vi "Case.vi"() -> ()   [LabVIEW 2013]
panel:
  out "Arbitary":bool
  out "Random":bool
  out "Sawtooth":bool
  out "Triangle":bool
  out "Square":bool
  out "Sine":bool
  in  "Triangle":bool
  in  "Random":bool
  in  "Arbitary":bool
  in  "Sine":bool
  in  "Square":bool
  in  "Sawtooth":bool
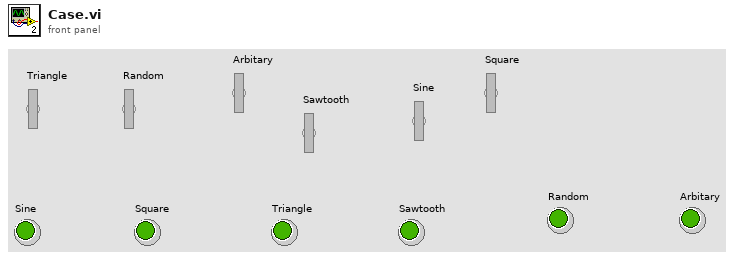
[diagram p1: front panel]
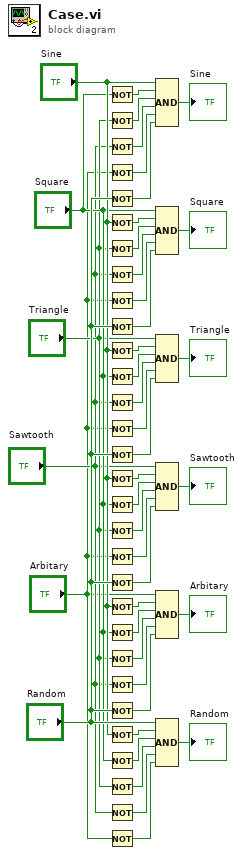
[diagram p0: block diagram]
diagram:
  n1 = Not(x="Square") -> (.not. x?=w42:bool)
  n2 = Not(x="Triangle") -> (.not. x?=w41:bool)
  n3 = Not(x="Sawtooth") -> (.not. x?=w40:bool)
  n4 = Not(x="Arbitary") -> (.not. x?=w39:bool)
  n5 = Not(x="Random") -> (.not. x?=w38:bool)
  n6 = Not(x="Sine") -> (.not. x?=w37:bool)
  n7 = Not(x="Triangle") -> (.not. x?=w36:bool)
  n8 = Not(x="Sawtooth") -> (.not. x?=w35:bool)
  n9 = Not(x="Arbitary") -> (.not. x?=w34:bool)
  n10 = Not(x="Random") -> (.not. x?=w33:bool)
  n11 = Not(x="Sine") -> (.not. x?=w32:bool)
  n12 = Not(x="Square") -> (.not. x?=w31:bool)
  n13 = Not(x="Sawtooth") -> (.not. x?=w30:bool)
  n14 = Not(x="Arbitary") -> (.not. x?=w29:bool)
  n15 = Not(x="Random") -> (.not. x?=w28:bool)
  n16 = Not(x="Sine") -> (.not. x?=w27:bool)
  n17 = Not(x="Square") -> (.not. x?=w26:bool)
  n18 = Not(x="Triangle") -> (.not. x?=w25:bool)
  n19 = Not(x="Arbitary") -> (.not. x?=w24:bool)
  n20 = Not(x="Random") -> (.not. x?=w23:bool)
  n21 = Not(x="Sine") -> (.not. x?=w22:bool)
  n22 = Not(x="Square") -> (.not. x?=w21:bool)
  n23 = Not(x="Triangle") -> (.not. x?=w20:bool)
  n24 = Not(x="Sawtooth") -> (.not. x?=w19:bool)
  n25 = Not(x="Random") -> (.not. x?=w18:bool)
  n26 = Not(x="Sine") -> (.not. x?=w17:bool)
  n27 = Not(x="Square") -> (.not. x?=w16:bool)
  n28 = Not(x="Triangle") -> (.not. x?=w15:bool)
  n29 = Not(x="Sawtooth") -> (.not. x?=w14:bool)
  n30 = Not(x="Arbitary") -> (.not. x?=w13:bool)
  n31 = Compound Arithmetic op=AND("Sine", w42, w41, w40, w39, w38) -> (→"Sine":bool)
  n32 = Compound Arithmetic op=AND("Square", w37, w36, w35, w34, w33) -> (→"Square":bool)
  n33 = Compound Arithmetic op=AND("Triangle", w32, w31, w30, w29, w28) -> (→"Triangle":bool)
  n34 = Compound Arithmetic op=AND("Sawtooth", w27, w26, w25, w24, w23) -> (→"Sawtooth":bool)
  n35 = Compound Arithmetic op=AND("Arbitary", w22, w21, w20, w19, w18) -> (→"Arbitary":bool)
  n36 = Compound Arithmetic op=AND("Random", w17, w16, w15, w14, w13) -> (→"Random":bool)
